vi "sigleAquire.vi"(11 "Shots":i32) -> (3 "TenAccumulate":cluster{"MassX":dbl[], "TenScans":sgl[]}(graph))   [LabVIEW 2013]
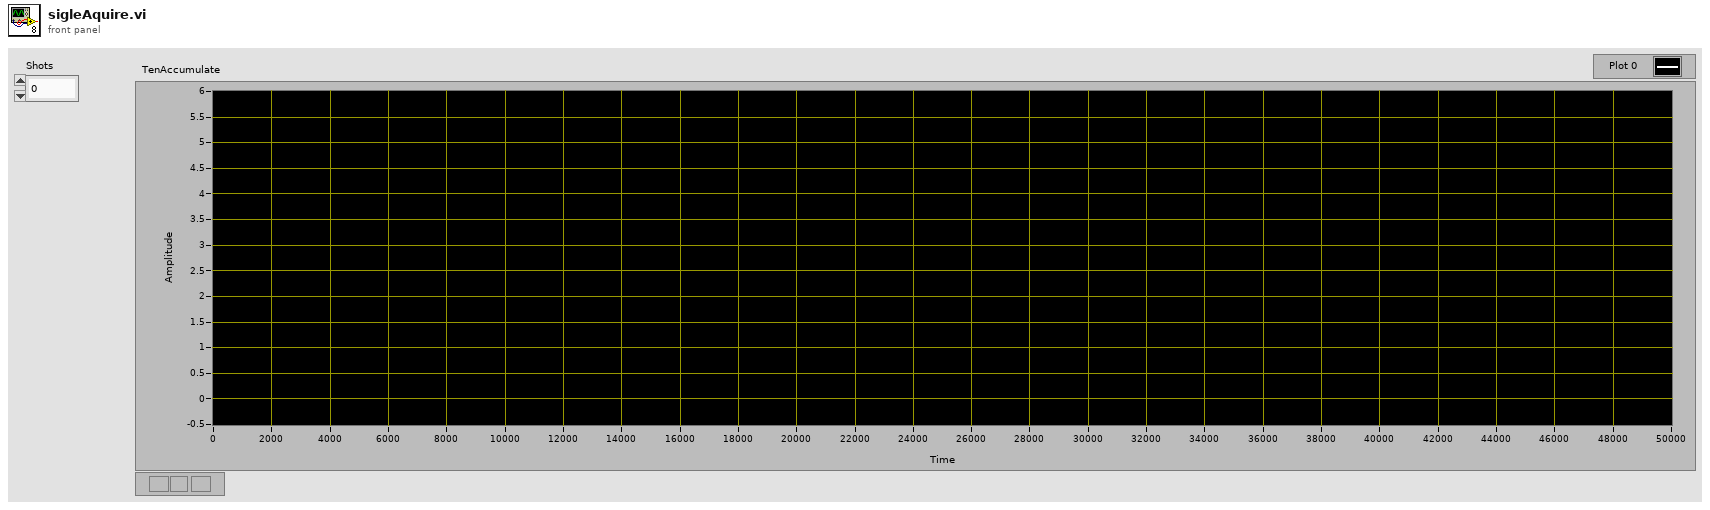
[diagram p1: front panel]
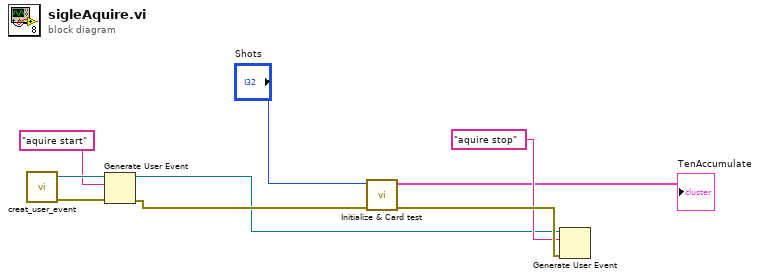
[diagram p0: block diagram]
diagram:
  n1 = call "creat_user_event.vi"() -> ("error out"=w8:errorcluster, "machine status"=w7:refnum<user-event>)  [unwired: 10 in]
  n2 = Generate User Event(user event=w7, event data cluster="aquire start" ("event data"), error in=w8) -> (user event out=w2:refnum<user-event>, error out=w5:errorcluster)  [unwired: 1 in]
  n3 = call "Initialize & Card test.vi"("error in (no error)"=w5, "ShotsPerPoint"="Shots") -> ("error out"=w4:errorcluster, "TenAccumulate"=→"TenAccumulate":cluster{"MassX":dbl[], "TenScans":sgl[]})  [unwired: 8 in]
  n4 = Generate User Event(user event=w2, event data cluster="aquire stop" ("event data"), error in=w4) -> ()  [unwired: 1 in, 2 out]
